vi "34401Aread.vi"(11 "Instrument Cluster":T1) -> (0 "Measurement value out":dbl)   [LabVIEW 2013]
uses:
  <vilib>/Utility/error.llb/DialogType.ctl
  <instrlib>/Agilent 34401/Public/Data/Read (Single Point).vi
  <instrlib>/Agilent 34401/Agilent 34401.lvlib
panel:
  out "after substring":string
  out "find instrument":string[](array[string])=["GPIB0::4::INSTR"]
  out "before substring":string
  out "Function (0: DC Voltage)":u16(ring) items=["DC Voltage", "AC Voltage", "2 - Wire Resistance", "4 - Wire Resistance", "DC Current", "AC Current", "Frequency", "Period", "Continuity", "Diode Checking", "VDC:VDC Ratio", "Temperature", "Capacitance"]
  out "Manual Range (1.00)":dbl=1.0 format="%_3f"
  out "Manual Resolution (5.5 Digits)":dbl(ring)=5.5 items=["4.5"=4.5, "5.5"=5.5, "6.5"=6.5]
  in  "VISA resource name":refnum<visa-resource-name>
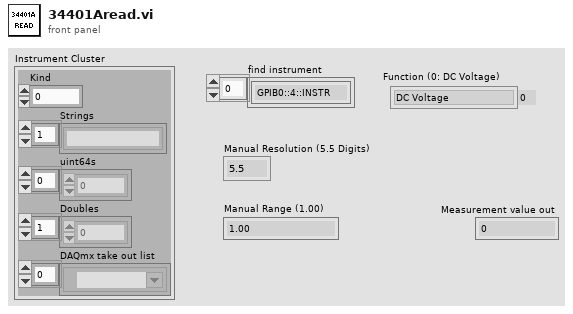
[diagram p1: front panel]
types:
  T1 = cluster{"Kind":u16, "Strings":string[], "uint64s":u64[], "Doubles":dbl[], "DAQmx take out list":refnum<k21>[]}
  T2 = cluster{"Baud Rate":u32, "Parity":u16, "Data Bits":u16}
  T3 = typedef "DialogType.ctl" = u16
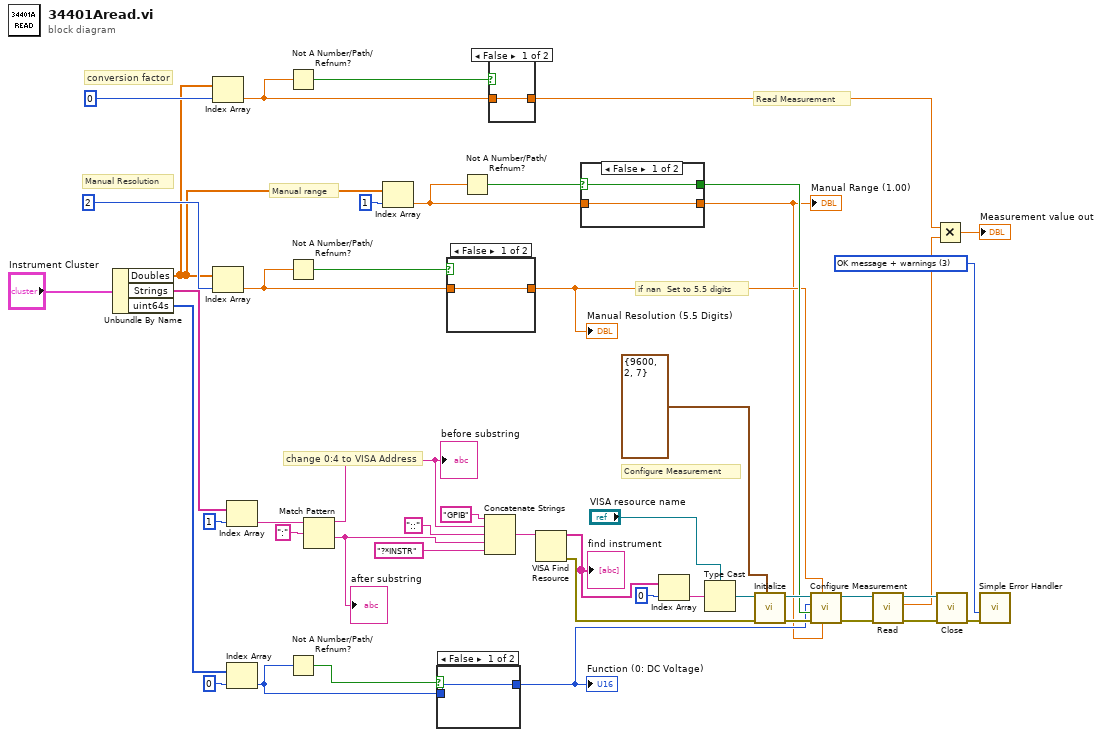
[diagram p0: block diagram]
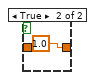
[diagram p2: hidden frame]
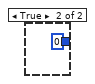
[diagram p3: hidden frame]
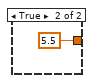
[diagram p4: hidden frame]
diagram:
  w40 = T3 3 items=["no dialog", "OK message", "continue or stop message", "OK message + warnings", "continue/stop + warnings"] ("type of dialog (OK msg:1)")
  # "change 0:4 to VISA Address"
  # "conversion factor"
  # "if nan  Set to 5.5 digits"
  # "Manual Resolution"
  # "Manual range"
  # "Read Measurement"
  # "Configure Measurement"
  n1 = Unbundle By Name("Instrument Cluster") -> ("Doubles"=w26:dbl[], "Strings"=w38:string[], "uint64s"=w22:u64[])
  n2 = Index Array(array=w26, index=0) -> (element=w16:dbl)
  n3 = Index Array(array=w26, index=2) -> (element=w30:dbl)
  n4 = Index Array(array=w38, index=1) -> (element=w12:string)
  n5 = Index Array(array=w22, index=0) -> (element=w19:u64)
  n6 = Not A Number/Path/Refnum?(number/path/refnum=w16) -> (NaN/Path/Refnum?=w17:bool)
  n7 = Not A Number/Path/Refnum?(number/path/refnum=w30) -> (NaN/Path/Refnum?=w31:bool)
  n8 = Not A Number/Path/Refnum?(number/path/refnum=w19) -> (NaN/Path/Refnum?=w21:bool)
  n9 = Match Pattern(string=w12, regular expression=":") -> (before substring=w8:string, after substring=w7:string)  [unwired: 1 in, 2 out]
  "before substring" <- w8
  "after substring" <- w7
  n10 = Index Array(array=w26, index=1) -> (element=w33:dbl)
  n11 = case shown="False" w21 {
    tunnel: [w48 0] -> w20
    tunnel: w19 -> [w48 _]
    frame False {
    }
    frame True {
    }
  }
  "Function (0: DC Voltage)" <- w20
  n12 = case shown="False" w31 {
    tunnel: [w50 5.5] -> w29
    tunnel: w30 -> [w50 _]
    frame False {
    }
    frame True {
    }
  }
  "Manual Resolution (5.5 Digits)" <- w29
  n13 = Not A Number/Path/Refnum?(number/path/refnum=w33) -> (NaN/Path/Refnum?=w36:bool)
  n14 = Concatenate Strings("GPIB", w8, "::", w7, "?*INSTR") -> (w5:string)
  n15 = case shown="False" w17 {
    tunnel: [w52 1.0] -> w15
    tunnel: w16 -> [w52 _]
    frame False {
    }
    frame True {
    }
  }
  n16 = VISA Find Resource(11:w5) -> (0:w1:errorcluster, 3:w4:string[])  [unwired: 2 in, 1 out]
  "find instrument" <- w4
  n17 = case shown="False" w36 {
    selector: w36 -> [w55 w56]
    tunnel: [w55 w56] -> w34
    tunnel: w33 -> [w54 _]
    tunnel: [w54 _] -> w18
    frame False {
    }
    frame True {
      # "if nan auto range True"
    }
  }
  "Manual Range (1.00)" <- w18
  n18 = Index Array(array=w4, index=0) -> (element=w2:string)
  n19 = Type Cast(type="VISA resource name", x=w2) -> (*(type *) &x=w13:refnum<visa-resource-name>)
  n20 = call <instrlib>:"Initialize.vi"("Serial Configuration"=T2 {"Baud Rate"=9600, "Parity"=2, "Data Bits"=7}, "error in (no error)"=w1, "VISA resource name"=w13) -> ("error out"=w35:errorcluster, "VISA resource name out"=w41:refnum<visa-resource-name>)  [unwired: 7 in]
  n21 = call <instrlib>:"Configure Measurement.vi"("Manual Range (1.00)"=w18, "Manual Resolution (5.5 Digits)"=w29, "error in (no error)"=w35, "Enable Auto Range (T: Enable)"=w34, "Function (0: DC Voltage)"=w20, "VISA resource name"=w41) -> ("error out"=w42:errorcluster, "VISA resource name out"=w43:refnum<visa-resource-name>)  [unwired: 4 in]
  n22 = call-poly <instrlib>:"Read.vi"("error in (no error)"=w42, "VISA resource name"=w43) -> ("error out"=w45:errorcluster, "Measurement"=w25:dbl, "VISA resource name out"=w44:refnum<visa-resource-name>)  [unwired: 7 in]
  n23 = Multiply(x=w15, y=w25) -> (x*y=→"Measurement value out":dbl)
  n24 = call <instrlib>:"Close.vi"("error in (no error)"=w45, "VISA resource name"=w44) -> ("error out"=w47:errorcluster)  [unwired: 9 in]
  n25 = call <vilib>:"Simple Error Handler.vi"("type of dialog (OK msg:1)"=w40, "error in (no error)"=w47) -> ()  [unwired: 3 in, 5 out]
